vi "QA-Trace.vi"(0 "trace string":string, 7 "trace integer":i32, 11 "error in (no error)":errorcluster) -> (15 "error out":errorcluster)   [LabVIEW 2020]
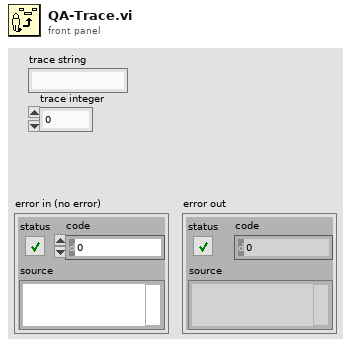
[diagram p1: front panel]
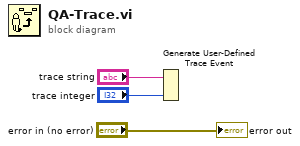
[diagram p0: block diagram]
diagram:
  n1 = Generate User-Defined Trace Event(1:"trace integer", 2:"trace string") -> ()
  "error out" <- "error in (no error)"
